vi "2DLev-Mar abx.vi"(0 "X":dbl[](array[numeric]) format="%.2f", 1 "Function":refnum<vi>, 2 "Y":dbl[](array[numeric]) format="%.2f", 3 "Coefficients":dbl[](array[numeric]) format="%.2f", 5 "W":dbl[](array[numeric]) format="%.2f") -> (6 "Alpha":dbl[][](array[numeric]) format="%.2f", 7 "Beta":dbl[](array[numeric]) format="%.2f", 8 "chiSqr":dbl format="%.2f")   [LabVIEW 2016]
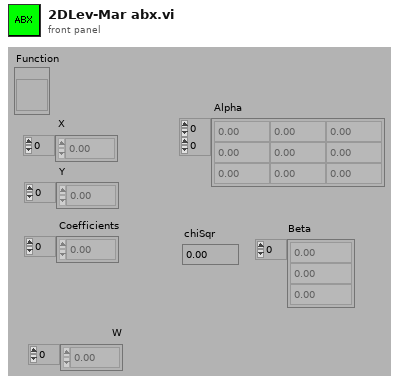
[diagram p1: front panel]
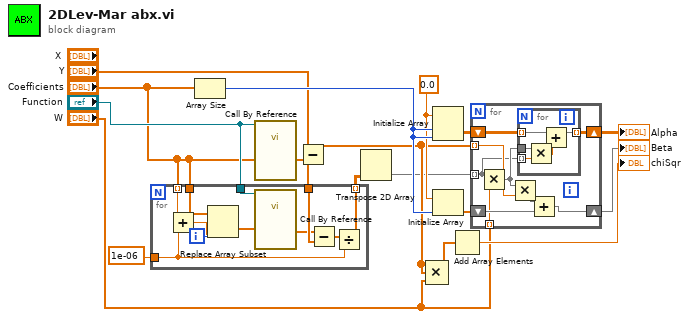
[diagram p0: block diagram]
diagram:
  w14 = 0.0
  n1 = Array Size(array="Coefficients") -> (size(s)=w17:i32)
  n2 = call-by-ref "?"(reference="Function", "Paramters"="Coefficients") -> ("Simulated Image"=w2:dbl[])  [unwired: 1 in, 2 out]
  n3 = for {
    tunnel: [w24] -> w4 mode=indexing
    tunnel: "Coefficients" -> [w25] mode=indexing
    tunnel: "Coefficients" -> [w23]
    tunnel: 1e-06 -> [w22]
    tunnel: w2 -> [w21]
    tunnel: "Function" -> [w20]
    i -> [w26]
    n4 = Add(x=w25, y=w22) -> (x+y=w27:dbl)
    n5 = Replace Array Subset(array=w23, new element=w27, index=w26) -> (w18:dbl[])
    n6 = call-by-ref "?"(reference=w20, "Paramters"=w18) -> ("Simulated Image"=w19:dbl[])  [unwired: 1 in, 2 out]
    n7 = Subtract(x=w19, y=w21) -> (x-y=w28:dbl[])
    n8 = Divide(x=w28, y=w22) -> (x/y=w24:dbl[])
  }
  n9 = Subtract(x="Y", y=w2) -> (x-y=w10:dbl[])
  n10 = Transpose 2D Array(2D array=w4) -> (transposed array=w6:dbl[][])
  n11 = Compound Arithmetic op=MULTIPLY(w10, w10, "W") -> (w9:dbl[])
  n12 = Initialize Array(w14, w17, w17) -> (w15:dbl[][])
  n13 = Initialize Array(w14, w17) -> (w16:dbl[])
  n14 = Add Array Elements(numeric array=w9) -> (sum=→"chiSqr":dbl)
  n15 = for {
    shift-right: [w35] -> w13
    shift-left: w16 -> [w37]
    shift-right: [w33] -> w12
    shift-left: w15 -> [w34]
    tunnel: w6 -> [w29] mode=indexing
    tunnel: w10 -> [w32] mode=indexing
    tunnel: "W" -> [w31] mode=indexing
    n16 = Multiply(x=w29, y=w31) -> (x*y=w30:dbl[])
    n17 = Multiply(x=w30, y=w32) -> (x*y=w36:dbl[])
    n18 = for {
      tunnel: w30 -> [w42]
      tunnel: w34 -> [w41] mode=indexing
      tunnel: [w39] -> w33 mode=indexing
      tunnel: w29 -> [w38] mode=indexing
      n19 = Multiply(x=w42, y=w38) -> (x*y=w40:dbl[])
      n20 = Add(x=w41, y=w40) -> (x+y=w39:dbl[])
    }
    n21 = Add(x=w36, y=w37) -> (x+y=w35:dbl[])
  }
  "Alpha" <- w12
  "Beta" <- w13
